vi "Display Main.vi"(8 "Stop Notifier In":refnum<notifier>, 11 "Display Actor in":refnum<class "Display Actor.lvclass">) -> (0 "Stop Notifier Out":refnum<notifier>, 3 "Display Actor out":refnum<class "Display Actor.lvclass">)   [LabVIEW 2024, in "Display Actor.lvclass"]
uses:
  Display Actor.lvclass
  Ancestor Class/Actor/System Actor/System Actor.lvclass/System Actor.ctl
  Ancestor Class/Actor/System Actor/Public Data/Read Actor Name.vi
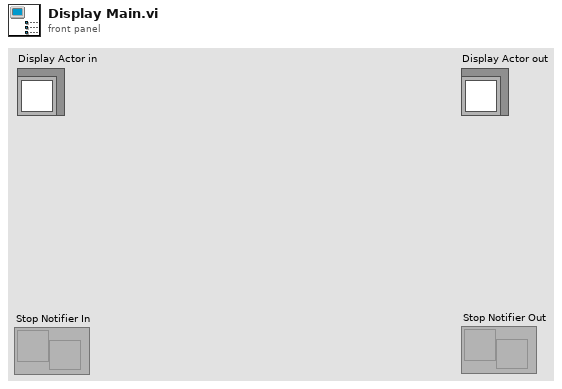
[diagram p1: front panel]
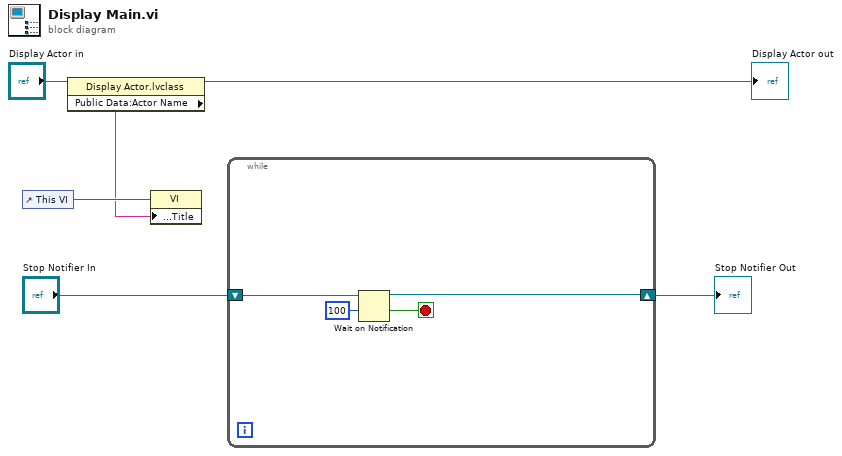
[diagram p0: block diagram]
diagram:
  n1 = control-ref of="This VI"() -> (w4:refnum<vi>)
  n2 = property class="Display Actor.lvclass"(reference="Display Actor in") -> (reference out=→"Display Actor out":refnum<class "Display Actor.lvclass">, "Public Data:Actor Name"=w3:string)  [unwired: 1 in, 1 out]
  n3 = property class="VI"(reference=w4, "Front Panel.Title"=w3) -> ()  [unwired: 1 in, 2 out]
  n4 = while {
    shift-right: [w9] -> w1
    shift-left: "Stop Notifier In" -> [w10]
    stop <- w7 stop-if-true
    n5 = Wait on Notification(notifier=w10, timeout in ms (-1)=100) -> (notifier out=w9:refnum<notifier>, timed out?=w7:bool)  [unwired: 2 in, 2 out]
  }
  "Stop Notifier Out" <- w1
